vi "IOS_Ephys_GCaMP_WhiskerTracking_Master.vi"() -> ()   [LabVIEW 2013]
uses:
  <vilib>/userdefined/High Color/IMAQdx.ctl
  <vilib>/vision/driver/IMAQdx.llb/IMAQdx Acquisition Mode.ctl
  <vilib>/vision/driver/IMAQdx.llb/IMAQdx Camera Control Mode.ctl
  <vilib>/vision/driver/IMAQdx.llb/IMAQdx Buffer Number Mode.ctl
  <vilib>/DAQmx/write.llb/DAQmx Write (Digital Bool 1Line 1Point).vi
  <vilib>/DAQmx/read.llb/DAQmx Read (Analog 1D Wfm NChan NSamp).vi
  <vilib>/DAQmx/write.llb/DAQmx Write (Digital 1D Bool NChan 1Samp 1Line).vi
  <vilib>/DAQmx/create/channels.llb/DAQmx Create Channel (DO-Digital Output).vi
  <vilib>/DAQmx/create/channels.llb/DAQmx Create Channel (CO-Pulse Generation-Frequency).vi
  <vilib>/DAQmx/configure/timing.llb/DAQmx Timing (Implicit).vi
  <vilib>/DAQmx/create/channels.llb/DAQmx Create Channel (AI-Voltage-Basic).vi
  <vilib>/DAQmx/configure/timing.llb/DAQmx Timing (Sample Clock).vi
  <vilib>/DAQmx/configure/trigger.llb/DAQmx Start Trigger (Digital Edge).vi
  <vilib>/DAQmx/miscellaneous.llb/DAQmx Fill In Error Info.vi
  <vilib>/vision/driver/NI_Vision_Acquisition_Software.lvlib
  <resource>/objmgr/imaqdx.rc
panel:
  in  "Exposure\nTime (microsec)":string="10000"
  out "Dropped Frame Table":string[][](table)
  out "Solenoids":bool[](array[boolean])
  out "Whisker Camera":bool
  out "Analog Data":bool
  out "Analog acquisition length":i32
  in  "Channel Labels":string[](array[string])=["Electrophysiology", "ForceSensor", "Solenoid_LeftPad", "Solenoid_RightPad", "Solenoid_Tail", "Solenoid_Auditory"]
  in  "physical channels":tag="Dev1/ai0:5, Dev1/ai7"
  in  "Whisker Cam ID":T1="cam2"
  in  "WebCam ID":T1="cam1"
  in  "Analog Acquisition Setup":cluster{"Analog Sampling Rate":u16}={"Analog Sampling Rate"=20000} {"Analog Sampling Rate" format="%0.0f"}
  in  "Camera Acquisition Setup":T2={"CBVCam Rate"=30, "WhiskerCam Rate"=150, "WebCam Rate"=15}
  out "Notes Size":i32=7
  out "Notes Reversed":string[](array[string])=["Experimenter", "Animal ID", "Imaged Hemisphere", "Solenoid Pressure", "Isoflurane time", "Session ID", "Amplifier Gain"]
  out "Notes Array":string[](array[string])=["Amplifier Gain", "Session ID", "Isoflurane time", "Solenoid Pressure", "Imaged Hemisphere", "Animal ID", "Experimenter"]
  in  "Session Notes:":T3={"Experimenter"="Kevin", "Animal ID"="T31", "Imaged Hemisphere"="Both", "Solenoid Pressure"="10", "Isoflurane time"="1200", "Session ID"="Habit1", "Amplifier Gain"="10000"}
  in  "Whisker Cam\nTrigger Source":tag="Dev1/ctr1"
  in  "CBV Cam\nTrigger Source":tag="Dev1/ctr0"
  in  "Left Pad":tag="Dev1/port0/line1"
  in  "Right Pad":tag="Dev1/port0/line0"
  in  "Auditory":tag="Dev1/port0/line3"
  in  "Tail":tag="Dev1/port0/line2"
  in  "Stim \nOffset (s)":dbl=15.0
  in  "Stim \nDuration (s)":dbl=0.1 step=0.1
  in  "Inter-Stim\nInterval (s)":dbl=30.0
  in  "Left Pad":dbl=1.0
  in  "Right Pad":dbl=1.0
  in  "Auditory":dbl
  in  "Tail":dbl
  in  "Target Path":path=path "A:/Turner Habituation" caption="Final saved file location"
  out "Dropped":u32(slide)=4 caption="Dropped Whisker\nCamera Frames" scale=0.0..50.0
  out "Current file name":string="170828_12_37_58"
  out "Actual WebCam Frame Rate":dbl(knob) scale=0.0..30.0
  out "WebCam":T4(plugin-control)
  out "CBV Camera":bool=TRUE
  out "Trial Time Elapsed (Min)":cluster{dbl, dbl}(slide)={0.5, 0.05364406000000001} scale=0.0..5.0
  in  "Recording Time (min)":dbl(knob)=5.0 min=0.5 max=10.0 step=0.5 scale=0.0..5.0 scale format="%#_2g"
  in  "Temp Path":path=path "C:/LabView Test Files" caption="Temporary path for\nstreamed data"
  out "Last CBV\nBuffer":i32=97
  in  "Stop":bool
  out "Actual CBVCam\nFrame Rate":dbl(knob)=30.019685039370078 scale=0.0..100.0
  out "Last Whisk\nBuffer":u32=488
  out "Actual WhiskCam\nFrame Rate":dbl(knob)=148.05583250249254 scale=0.0..300.0
  # "Dropped\nIndex"
  # "# Dropped"
  # "File Settings:"
  # "Right Pad"
  # "Left Pad"
  # "Tail"
  # "Auditory"
  # "Stimulation Settings:"
  # "Stim. Ratios:"
  # "Output Channels:"
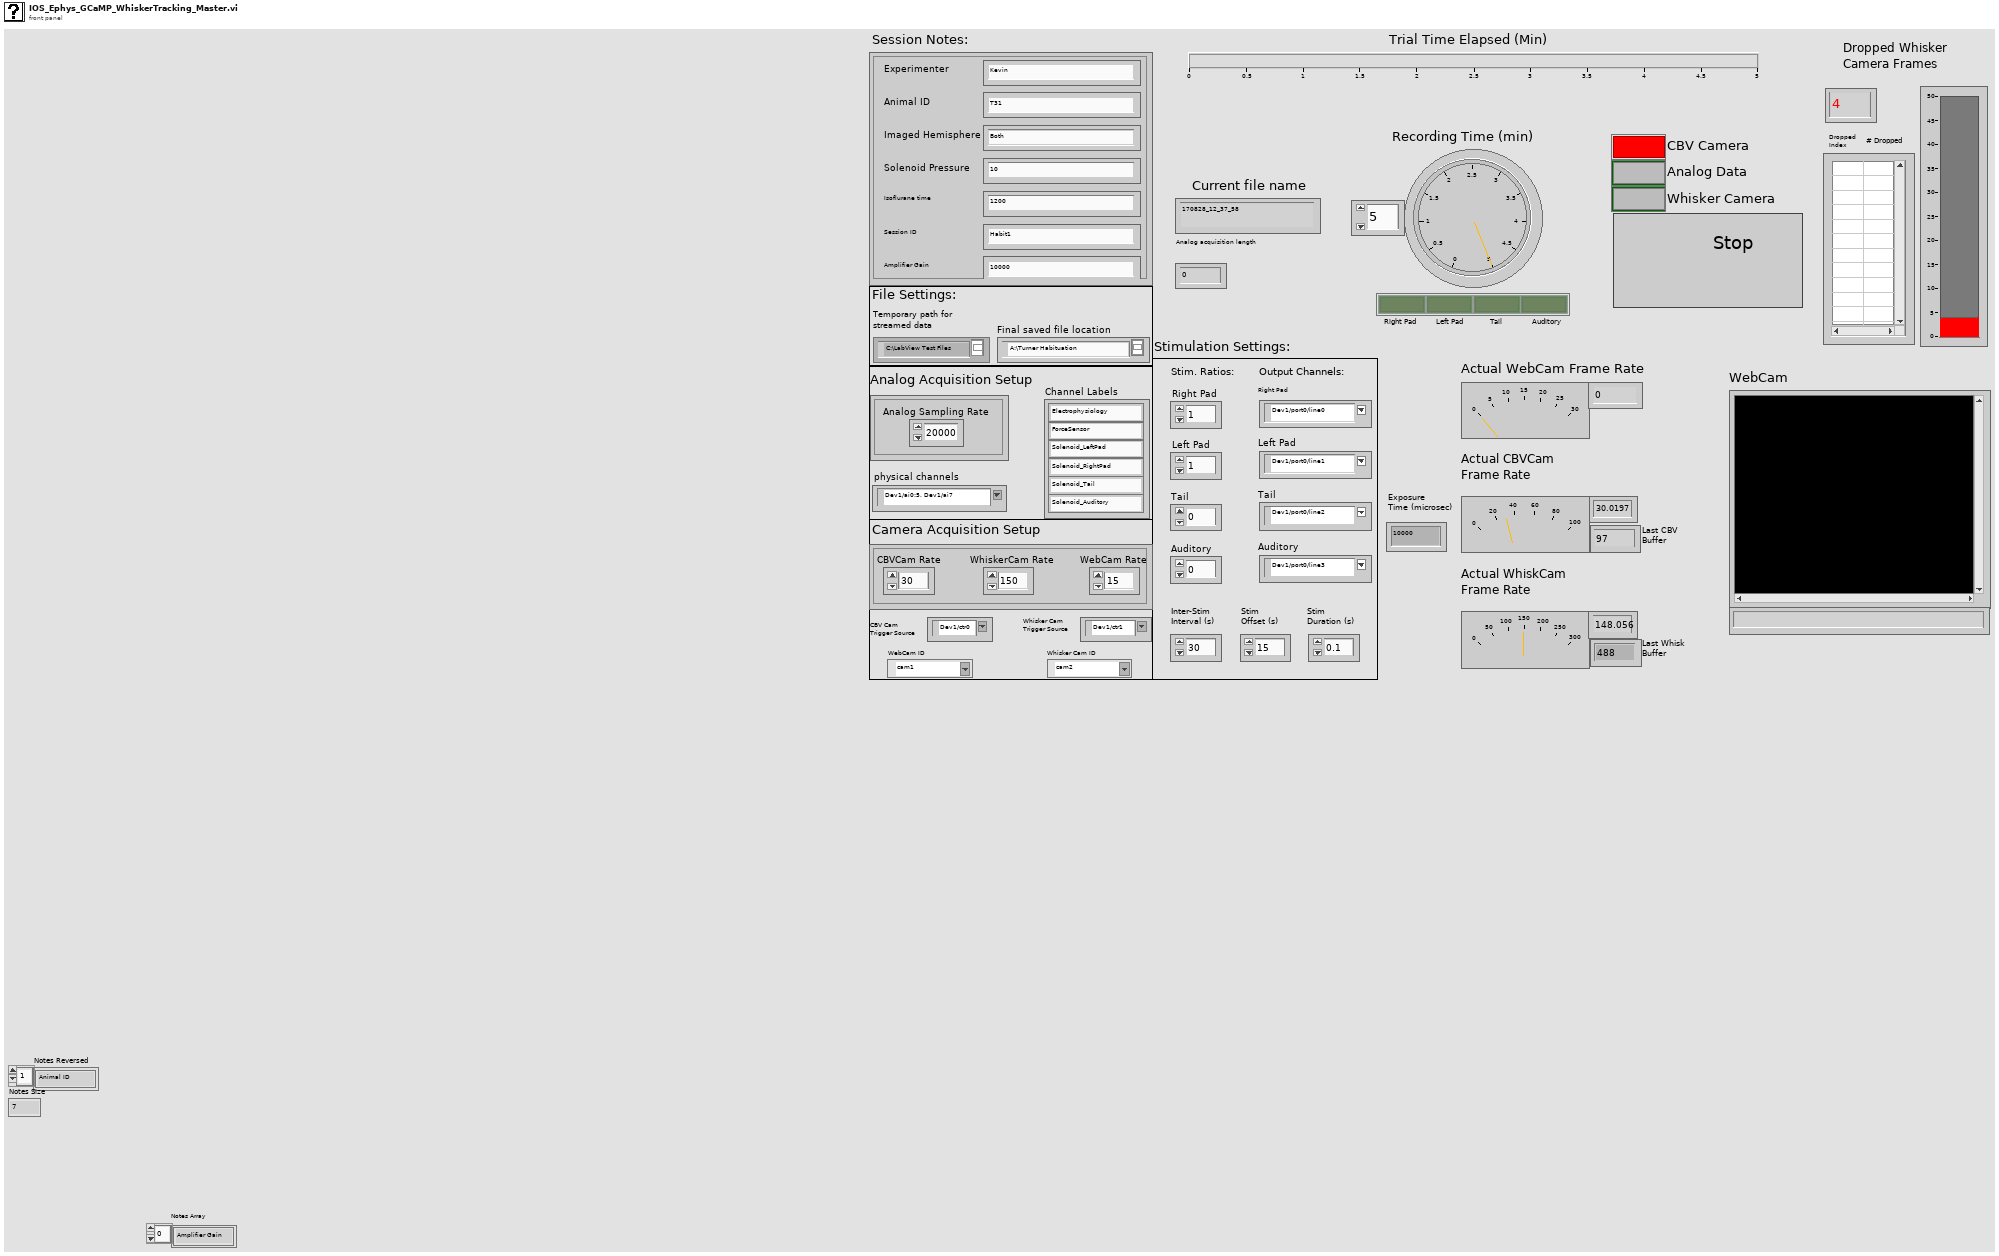
[diagram p1: front panel]
types:
  T1 = typedef "IMAQdx.ctl" = refnum<k21>
  T2 = cluster{"CBVCam Rate":u16, "WhiskerCam Rate":u16, "WebCam Rate":u16}
  T3 = cluster{"Experimenter":string, "Animal ID":string, "Imaged Hemisphere":string, "Solenoid Pressure":string, "Isoflurane time":string, "Session ID":string, "Amplifier Gain":string}
  T4 = typedef "IMAQ Image.ctl" = refnum<image>
  T5 = enum16{"open", "open or create", "create or replace", "create", "open (read-only)"}
  T6 = typedef "Image Type" = u32
  T7 = typedef "NI_Vision_Acquisition_Software.lvlib/IMAQdx Camera Control Mode.ctl" = enum32{"Controller", "Listener"}
  T8 = enum16{"open", "replace", "create", "open or create", "replace or create", "replace or create with confirmation"}
  T9 = typedef "NI_Vision_Acquisition_Software.lvlib/IMAQdx Acquisition Mode.ctl" = enum32{"One Shot", "Continuous"}
  T10 = typedef "IMAQ AVI2 Refnum.ctl" = refnum<k20>
  T11 = enum16{"big-endian, network order", "native, host order", "little-endian"}
  T12 = typedef "NI_Vision_Acquisition_Software.lvlib/IMAQdx Buffer Number Mode.ctl" = enum32{"Next", "Last", "Buffer Number"}
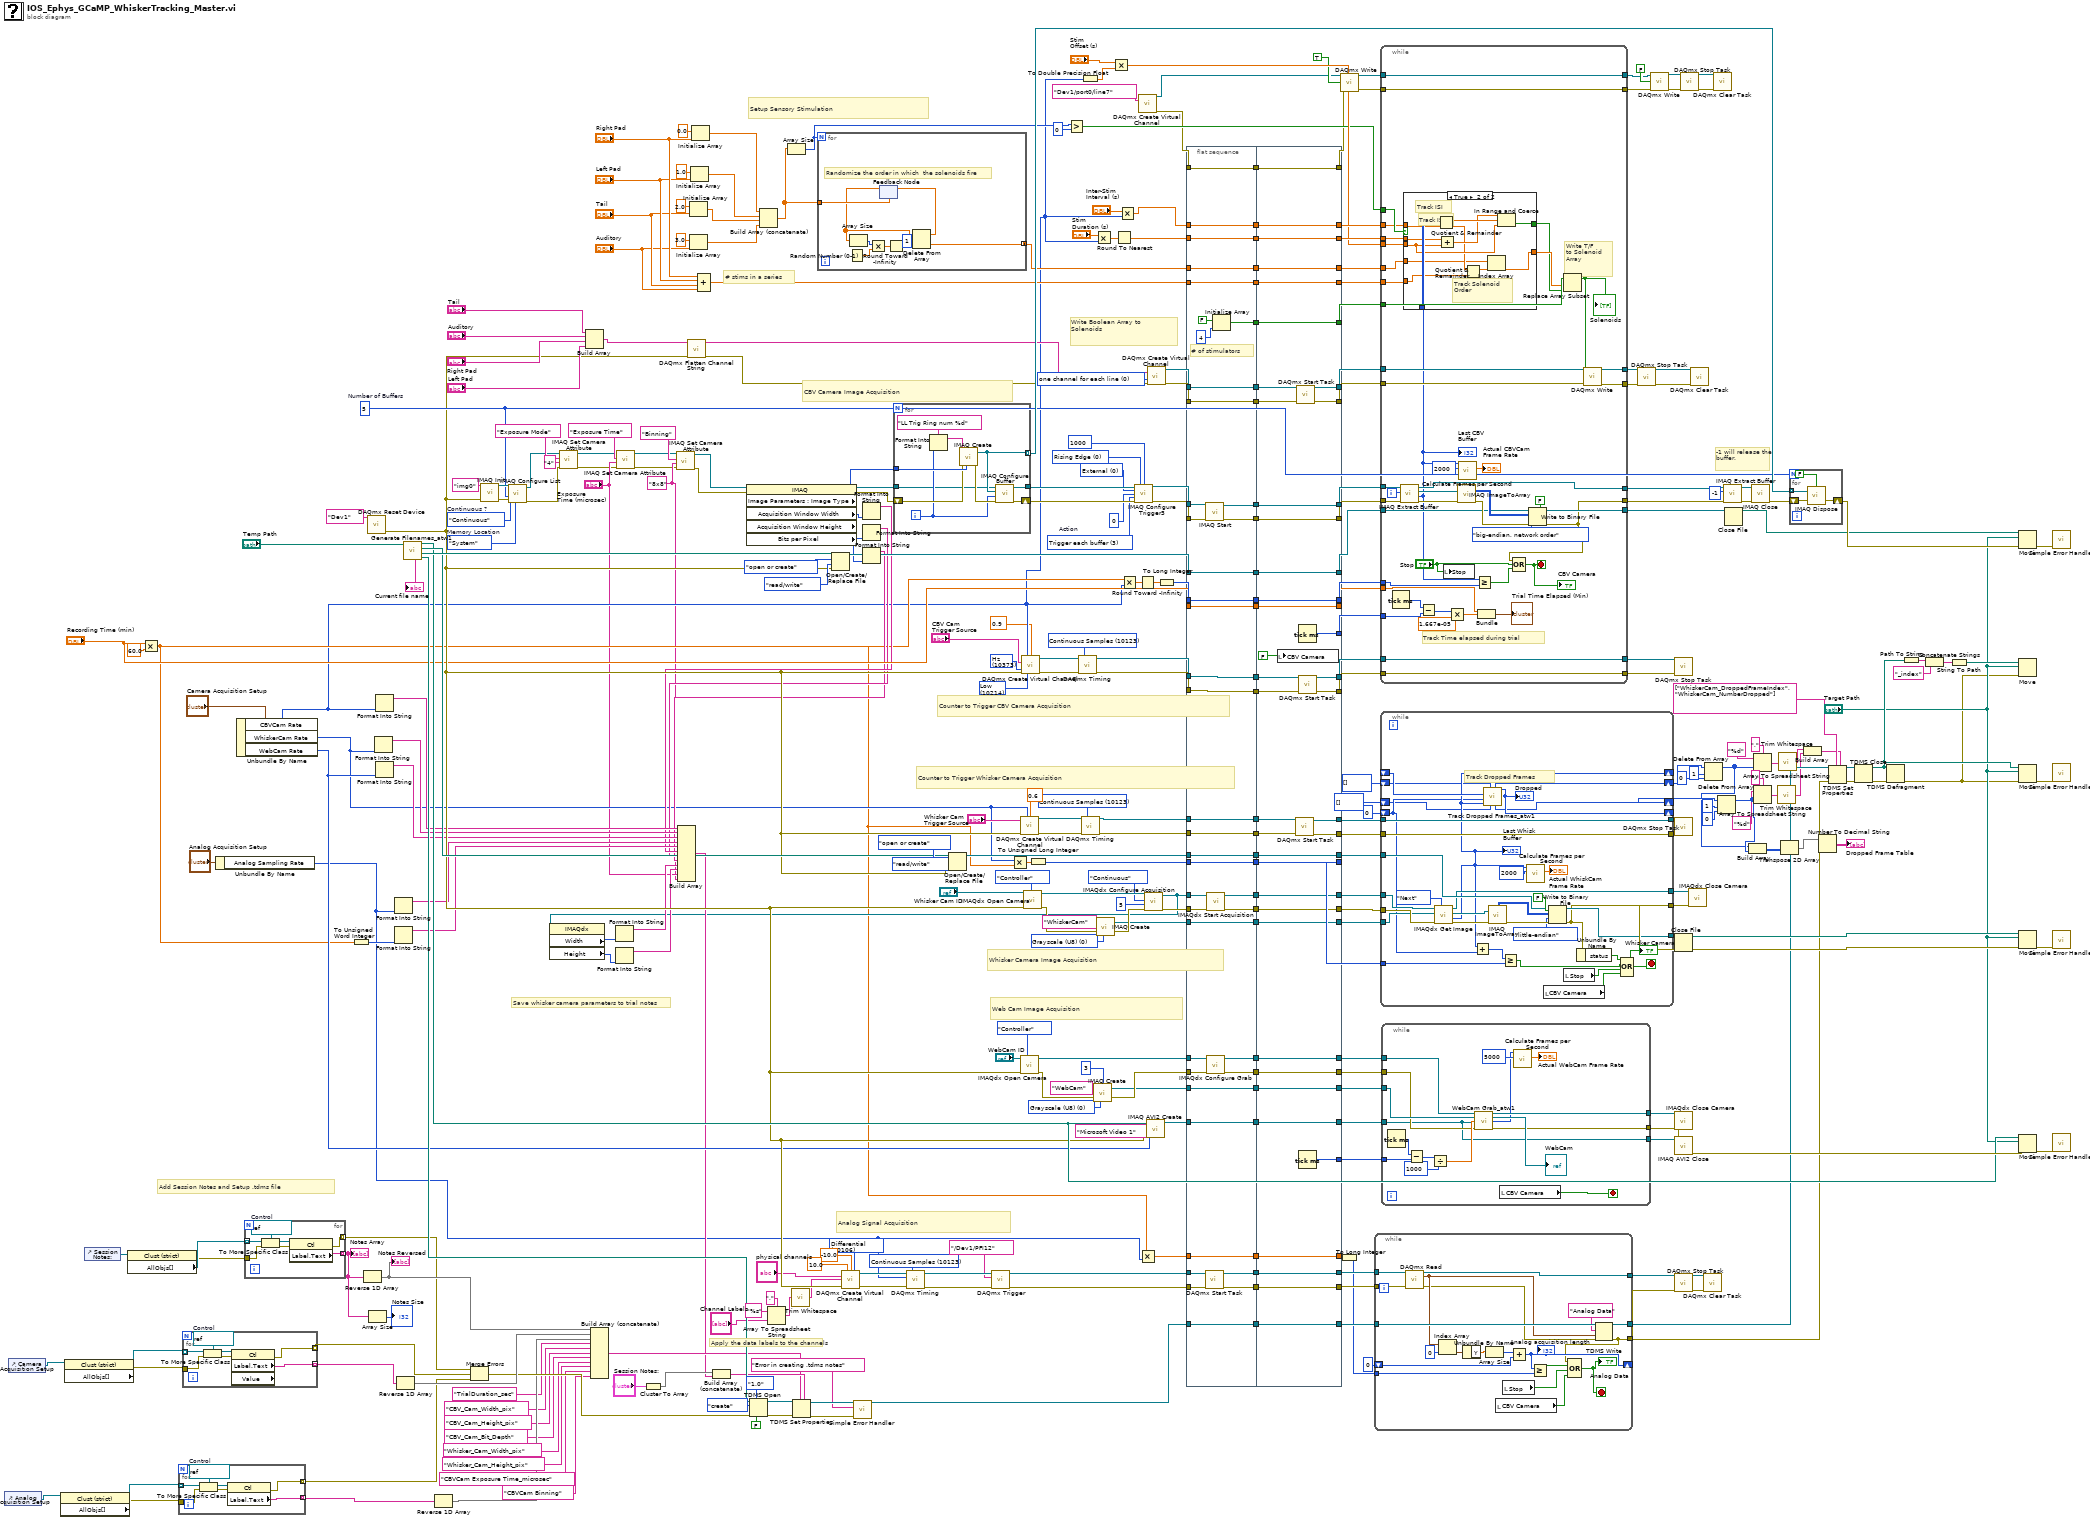
[diagram p0: block diagram]
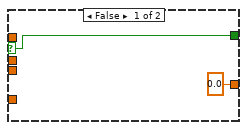
[diagram p2: hidden frame]
diagram:
  w15 = "8x8" ("Attribute Value")
  w189 = 0 items=["one channel for each line", "one channel for all lines"] ("line grouping")
  w248 = 10123 items=["Finite Samples"=10178, "Continuous Samples"=10123, "Hardware Timed Single Point"=12522] ("sample mode")
  w251 = 10106 items=["default"=-1, "RSE"=10083, "NRSE"=10078, "Differential"=10106, "Pseudodifferential"=12529] ("input terminal configuration")
  w305 = T6 0 items=["Grayscale (U8)", "Grayscale (I16)", "Grayscale (SGL)", "Complex (CSG)", "RGB (U32)", "HSL (U32)", "RGB (U64)", "Grayscale (U16)"] ("Image Type")
  w327 = u32 0 items=["Rising Edge", "Falling Edge"] ("Trigger Polarity")
  w330 = u32 0 items=["External"=0, "RTSI"=1, "ISO In"=2, "Scaled Encoder"=5] ("Trigger Type")
  w321 = 10123 items=["Finite Samples"=10178, "Continuous Samples"=10123, "Hardware Timed Single Point"=12522] ("sample mode")
  w324 = 10373 items=["Hz"=10373] ("units")
  w325 = 10214 items=["High"=10192, "Low"=10214] ("idle state")
  w156 = u32 5  # Number of Buffers
  w328 = u32 3 items=["Disabled", "Trigger start of acquisition", "Trigger start of each buffer list", "Trigger each buffer", "Trigger each line (linescan)", "Trigger end of acquisition"]  # Action
  w335 = enum16{"System", "Onboard"}."System"  # Memory Location
  w334 = enum16{"One-Shot", "Continuous"}."Continuous"  # Continuous ?
  w343 = 10123 items=["Finite Samples"=10178, "Continuous Samples"=10123, "Hardware Timed Single Point"=12522] ("sample mode")
  w350 = T6 0 items=["Grayscale (U8)", "Grayscale (I16)", "Grayscale (SGL)", "Complex (CSG)", "RGB (U32)", "HSL (U32)", "RGB (U64)", "Grayscale (U16)"] ("Image Type")
  # "Save whisker camera parameters to trial notes"
  # "Apply the data labels to the channels"
  # "Setup Sensory Stimulation"
  # "CBV Camera Image Acquisition"
  # "Counter to Trigger CBV Camera Acquisition"
  # "Counter to Trigger Whisker Camera Acquisition"
  # "Whisker Camera Image Acquisition"
  # "Web Cam Image Acquisition"
  # "Add Session Notes and Setup .tdms file"
  # "Analog Signal Acquisition"
  # "Write Boolean Array to \nSolenoids"
  # "# stims in a series"
  # "-1 will release the buffer."
  n1 = control-ref of="Analog Acquisition Setup"() -> (w116:refnum<vi>)
  n2 = control-ref of="Camera Acquisition Setup"() -> (w117:refnum<vi>)
  n3 = property class="Clust (strict)"(reference=w116) -> (error out=w114:errorcluster, "AllObjs[]"=w115:refnum<vi>[])  [unwired: 1 in, 1 out]
  n4 = property class="Clust (strict)"(reference=w117) -> (error out=w139:errorcluster, "AllObjs[]"=w138:refnum<vi>[])  [unwired: 1 in, 1 out]
  n5 = control-ref of="Session Notes:"() -> (w142:refnum<vi>)
  n6 = property class="Clust (strict)"(reference=w142) -> (error out=w145:errorcluster, "AllObjs[]"=w146:refnum<vi>[])  [unwired: 1 in, 1 out]
  n7 = Multiply(x="Recording Time (min)", y=60.0) -> (x*y=w49:dbl)
  n8 = for {
    tunnel: [w362] -> w112 mode=indexing
    tunnel: w115 -> [w361] mode=indexing
    tunnel: w114 -> [w360]
    tunnel: [w358] -> w113 mode=indexing
    w363 = refnum<vi> refnum  # Control
    n9 = To More Specific Class(target class=w363, reference=w361, error in=w360) -> (specific class reference=w364:refnum<vi>, error out=w359:errorcluster)
    n10 = property class="Ctl"(reference=w364, error in=w359) -> (error out=w358:errorcluster, "Label.Text"=w362:string)  [unwired: 1 out]
  }
  n11 = for {
    tunnel: [w369] -> w140 mode=indexing
    tunnel: w138 -> [w368] mode=indexing
    tunnel: w139 -> [w367]
    tunnel: [w365] -> w123 mode=indexing
    w370 = refnum<vi> refnum  # Control
    n12 = To More Specific Class(target class=w370, reference=w368, error in=w367) -> (specific class reference=w371:refnum<vi>, error out=w366:errorcluster)
    n13 = property class="Ctl" props=["Label", "Text", "Value"](reference=w371, error in=w366) -> (error out=w365:errorcluster, "Label.Text"=w369:string)  [unwired: 2 out]
  }
  n14 = Unbundle By Name("Analog Acquisition Setup") -> ("Analog Sampling Rate"=w55:u16)
  n15 = Unbundle By Name("Camera Acquisition Setup") -> ("CBVCam Rate"=w23:u16, "WhiskerCam Rate"=w50:u16, "WebCam Rate"=w109:u16)
  n16 = for {
    tunnel: [w376] -> w144 mode=indexing
    tunnel: w146 -> [w375] mode=indexing
    tunnel: w145 -> [w374]
    tunnel: [w372] -> w124 mode=indexing
    w377 = refnum<vi> refnum  # Control
    n17 = To More Specific Class(target class=w377, reference=w375, error in=w374) -> (specific class reference=w378:refnum<vi>, error out=w373:errorcluster)
    n18 = property class="Ctl"(reference=w378, error in=w373) -> (error out=w372:errorcluster, "Label.Text"=w376:string)  [unwired: 1 out]
  }
  "Notes Array" <- w144
  n19 = To Unsigned Word Integer(number=w49) -> (unsigned 16bit integer=w91:u16)
  n20 = Reverse 1D Array(array=w144) -> (reversed array=w129:string[])
  "Notes Reversed" <- w129
  n21 = call <vilib>:"DAQmx Reset Device.vi"("device in"=tag "Dev1") -> ("error out"=w141:errorcluster)  [unwired: 14 in]
  n22 = Array Size(array=w144) -> (size(s)=→"Notes Size":i32)
  n23 = Format Into String(w50) -> (resulting string=w107:string)  [unwired: 3 in, 1 out]
  n24 = Format Into String(w23) -> (resulting string=w108:string)  [unwired: 3 in, 1 out]
  n25 = Format Into String(w109) -> (resulting string=w106:string)  [unwired: 3 in, 1 out]
  n26 = Format Into String(w55) -> (resulting string=w105:string)  [unwired: 3 in, 1 out]
  n27 = Format Into String(w91) -> (resulting string=w93:string)  [unwired: 3 in, 1 out]
  n28 = Reverse 1D Array(array=w140) -> (reversed array=w128:string[])
  n29 = call "Generate Filenames_atw1.vi"("path"="Temp Path") -> ("TDMS Path"=w135:path, "Dalsa Path"=w313:path, "Basler Path"=w308:path, "WebCam Path"=w213:path, "Analog file name"=→"Current file name":string)  [unwired: 5 in, 1 out]
  n30 = Reverse 1D Array(array=w112) -> (reversed array=w111:string[])
  n31 = Merge Errors(w124, w123, w113) -> (w122:errorcluster)
  n32 = call <vilib>:"IMAQ Init.vi"("error in (no error)"=w141, "Interface Name"="img0") -> ("error out"=w341:errorcluster, "IMAQ Session Out"=w342:refnum<k11>)  [unwired: 8 out]
  n33 = call <vilib>:"IMAQ Configure List.vi"("Memory Location"=w335, "error in (no error)"=w341, "Number of buffers"=w156, "Continuous?"=w334, "IMAQ Session In"=w342) -> ("error out"=w14:errorcluster, "IMAQ Session Out"=w10:refnum<k11>)  [unwired: 1 in, 4 out]
  n34 = call <vilib>:"IMAQ Set Camera Attribute.vi"("error in (no error)"=w14, "Attribute Value"="4", "Camera Attribute"="Exposure Mode", "IMAQ Session In"=w10) -> ("error out"=w13:errorcluster, "IMAQ Session Out"=w9:refnum<k11>)  [unwired: 4 in]
  n35 = Build Array("Tail", "Auditory", "Right Pad", "Left Pad") -> (w148:tag[])
  n36 = Build Array (concatenate)(w129, w128, w111, "TrialDuration_sec", "CBV_Cam_Width_pix", "CBV_Cam_Height_pix", "CBV_Cam_Bit_Depth", "Whisker_Cam_Width_pix", "Whisker_Cam_Height_pix", "CBVCam Exposure Time_microsec" ("element"), "CBVCam Binning" ("element")) -> (w126:string[])
  n37 = call <vilib>:"IMAQ Set Camera Attribute.vi"("error in (no error)"=w13, "Attribute Value"="Exposure\nTime (microsec)", "Camera Attribute"="Exposure Time", "IMAQ Session In"=w9) -> ("error out"=w12:errorcluster, "IMAQ Session Out"=w8:refnum<k11>)  [unwired: 4 in]
  n38 = Cluster To Array(cluster="Session Notes:") -> (array=w136:string[])
  n39 = call <vilib>:"IMAQ Set Camera Attribute.vi"("error in (no error)"=w12, "Attribute Value"=w15, "Camera Attribute"="Binning", "IMAQ Session In"=w8) -> ("error out"=w11:errorcluster, "IMAQ Session Out"=w7:refnum<k11>)  [unwired: 4 in]
  n40 = call <vilib>:"DAQmx Flatten Channel String.vi"("names in"=w148, "error in"=w141) -> ("names out"=w153:string, "error out"=w147:errorcluster)  [unwired: 12 in]
  n41 = Initialize Array(2.0 ("element"), "Tail") -> (w194:dbl[])
  n42 = Initialize Array(3.0 ("element"), "Auditory") -> (w193:dbl[])
  n43 = Initialize Array(1.0 ("element"), "Left Pad") -> (w195:dbl[])
  n44 = Initialize Array(0.0 ("element"), "Right Pad") -> (w196:dbl[])
  n45 = Compound Arithmetic op=ADD("Right Pad", "Left Pad", "Tail", "Auditory") -> (w173:dbl)
  n46 = property class="IMAQ"(reference=w7, error in=w11) -> (reference out=w25:refnum<k11>, error out=w24:errorcluster, "Image Parameters : Image Type"=w336:u32, "Acquisition Window Width"=w88:u32, "Acquisition Window Height"=w87:u32, "Bits per Pixel"=w86:u32)
  n47 = TDMS Open(6:FALSE ("disable buffering? (T)"), 7:enum16{"1.0", "2.0"}."1.0" ("file format version (2.0)"), 8:w122, 10:T5."create" ("operation (0:open)"), 11:w135) -> (0:w130:errorcluster, 3:w131:refnum<k34>)  [unwired: 2 in]
  n48 = Build Array (concatenate)(w196, w195, w194, w193) -> (w192:dbl[])
  n49 = Array To Spreadsheet String(delimiter (Tab)=",", array="Channel Labels", 3:"%s" ("format string")) -> (spreadsheet string=w97:string)
  n50 = Array Size(array=w192) -> (size(s)=w102:i32)
  n51 = call <vilib>:"Trim Whitespace.vi"("string"=w97) -> ("trimmed string"=w96:string)  [unwired: 1 in]
  n52 = for {
    N: w102 -> [_]
    tunnel: w192 -> [w382]
    tunnel: [w379] -> w170 mode=concatenating
    # "Randomize the order in which  the solenoids fire"
    n53 = Random Number (0-1)() -> (number: 0 to 1=w386:dbl)
    n54 = feedback #1(w382) -> (w381:dbl[])
    n55 = Array Size(array=w381) -> (size(s)=w387:i32)
    n56 = Multiply(x=w387, y=w386) -> (x*y=w385:dbl)
    n57 = Round Toward -Infinity(1:w385) -> (0:w384:dbl)
    n58 = Delete From Array(array=w381, length=1, index=w384) -> (deleted portion=w379:dbl[], array with subset deleted=w380:dbl[])
    n59 = feedback-in #1(w380) -> ()
  }
  n60 = Open/Create/Replace File(file path (use dialog)=w313, error in=w141, operation (0:open)=T8."open or create", access (0:read/write)=enum16{"read/write", "read-only", "write-only"}."read/write") -> (refnum out=w252:refnum<file>)  [unwired: 2 in, 2 out]
  n61 = call-poly <vilib>:"DAQmx Create Virtual Channel.vi"("maximum value"=10.0, "minimum value"=-10.0, "input terminal configuration"=w251, "physical channels"="physical channels", "name to assign"=w96, "error in"=w141) -> ("task out"=w250:refnum<k21>, "error out"=w249:errorcluster)  [unwired: 8 in]
  n62 = Format Into String(w88) -> (resulting string=w85:string)  [unwired: 3 in, 1 out]
  n63 = Format Into String(w87) -> (resulting string=w84:string)  [unwired: 3 in, 1 out]
  n64 = Format Into String(w86) -> (resulting string=w83:string)  [unwired: 3 in, 1 out]
  n65 = for {
    N: w156 -> [_]
    tunnel: [w397] -> w332
    tunnel: w336 -> [w395]
    shift-right: [w396] -> w331
    shift-left: w24 -> [w394]
    tunnel: [w389] -> w333 mode=indexing
    tunnel: w25 -> [w388]
    i -> [w390]
    n66 = Format Into String(format string="LL Trig Ring num %d", w390) -> (resulting string=w392:string)  [unwired: 2 in, 1 out]
    n67 = call "IMAQ Create"("Image Name"=w392, "Image Type"=w395, "error in (no error)"=w394) -> ("New Image"=w389:T4, "error out"=w393:errorcluster)  [unwired: 1 in, 1 out]
    n68 = call <vilib>:"IMAQ Configure Buffer.vi"("error in (no error)"=w393, "Buffer Number"=w390, "Image In"=w389, "IMAQ Session In"=w388) -> ("error out"=w396:errorcluster, "IMAQ Session Out"=w397:refnum<k11>)  [unwired: 2 in, 4 out]
  }
  n69 = call-poly <vilib>:"DAQmx Timing.vi"("task/channels in"=w250, "sample mode"=w248, "rate"=w55, "error in"=w249) -> ("task out"=w247:refnum<k21>, "error out"=w246:errorcluster)  [unwired: 10 in]
  n70 = Open/Create/Replace File(file path (use dialog)=w308, error in=w141, operation (0:open)=T8."open or create", access (0:read/write)=enum16{"read/write", "read-only", "write-only"}."read/write") -> (refnum out=w271:refnum<file>)  [unwired: 2 in, 2 out]
  n71 = call-poly <vilib>:"DAQmx Trigger.vi"("task/channels in"=w247, "source"=tag "/Dev1/PFI12", "error in"=w246) -> ("task out"=w244:refnum<k21>, "error out"=w243:errorcluster)  [unwired: 11 in]
  n72 = Multiply(x=w50, y=w49) -> (x*y=w48:dbl)
  n73 = call <vilib>:"IMAQdx Open Camera.vi"("Camera Control Mode"=IMAQdx_Camera_Control_Mode."Controller", "error in"=w141, "Session In"="WebCam ID") -> ("error out"=w301:errorcluster, "Session Out"=w299:T1)  [unwired: 7 in]
  n74 = call-poly <vilib>:"DAQmx Create Virtual Channel.vi"("frequency"=w50, "duty cycle"=0.6, "counter"="Whisker Cam\nTrigger Source", "error in"=w141) -> ("task out"=w345:refnum<k21>, "error out"=w344:errorcluster)  [unwired: 10 in]
  n75 = call-poly <vilib>:"DAQmx Create Virtual Channel.vi"("frequency"=w23, "duty cycle"=0.9, "counter"="CBV Cam\nTrigger Source", "units"=w324, "error in"=w141, "idle state"=w325) -> ("task out"=w323:refnum<k21>, "error out"=w322:errorcluster)  [unwired: 8 in]
  n76 = call <vilib>:"IMAQdx Open Camera.vi"("Camera Control Mode"=IMAQdx_Camera_Control_Mode."Controller", "error in"=w141, "Session In"="Whisker Cam ID") -> ("error out"=w353:errorcluster, "Session Out"=w356:T1)  [unwired: 7 in]
  n77 = To Unsigned Long Integer(number=w48) -> (unsigned 32bit integer=w47:u32)
  n78 = Greater?(x=w102, y=0) -> (0:w100:bool)
  n79 = call-poly <vilib>:"DAQmx Timing.vi"("task/channels in"=w323, "sample mode"=w321, "error in"=w322) -> ("task out"=w234:refnum<k21>, "error out"=w232:errorcluster)  [unwired: 11 in]
  n80 = call-poly <vilib>:"DAQmx Timing.vi"("task/channels in"=w345, "sample mode"=w343, "error in"=w344) -> ("task out"=w230:refnum<k21>, "error out"=w228:errorcluster)  [unwired: 11 in]
  n81 = To Double Precision Float(number=w23) -> (double precision float=w154:dbl)
  n82 = call "IMAQ Create"("Border Size"=3, "Image Name"="WebCam", "Image Type"=w305, "error in (no error)"=w301) -> ("New Image"=w298:T4, "error out"=w300:errorcluster)  [unwired: 1 in]
  n83 = Multiply(x="Stim \nDuration (s)", y=w23) -> (x*y=w164:dbl)
  n84 = call "IMAQ Create"("Image Name"="WhiskerCam", "Image Type"=w350, "error in (no error)"=w353) -> ("New Image"=w73:T4, "error out"=w351:errorcluster)  [unwired: 2 in]
  n85 = Multiply(x="Stim \nOffset (s)", y=w154) -> (x*y=w155:dbl)
  n86 = Round To Nearest(number=w164) -> (nearest integer value=w163:dbl)
  n87 = Multiply(x="Inter-Stim\nInterval (s)", y=w23) -> (x*y=w177:dbl)
  n88 = Multiply(x=w49, y=w23) -> (x*y=w310:dbl)
  n89 = call <vilib>:"IMAQ Configure Trigger3.vi"("IMAQ Session In"=w332, "Polarity"=w327, "Frame timeout (ms)"=u32 1000 ("Frame Timeout (ms)"), "Type"=w330, "Line Number"=u32 0 ("Trigger Line Number"), "Action"=w328, "error in (no error)"=w331) -> ("IMAQ Session Out"=w270:refnum<k11>, "error out"=w269:errorcluster)  [unwired: 2 in, 5 out]
  n90 = call-poly <vilib>:"DAQmx Create Virtual Channel.vi"("lines"=tag "Dev1/port0/line7") -> ("task out"=w39:refnum<k21>, "error out"=w42:errorcluster)  [unwired: 13 in]
  n91 = Round Toward -Infinity(1:w310) -> (0:w309:dbl)
  n92 = Multiply(x=w49, y=w55) -> (x*y=w54:dbl)
  n93 = call <vilib>:"IMAQdx Configure Acquisition.vi"("error in"=w351, "Number of Buffers"=u32 5, "Continuous?"=IMAQdx_Acquisition_Mode."Continuous", "Session In"=w356) -> ("error out"=w280:errorcluster, "Session Out"=w74:T1)  [unwired: 6 in]
  n94 = property class="IMAQdx"(reference=w74) -> ("Width"=w90:u32, "Height"=w89:u32)  [unwired: 1 in, 2 out]
  n95 = Format Into String(w90) -> (resulting string=w82:string)  [unwired: 3 in, 1 out]
  n96 = Format Into String(w89) -> (resulting string=w81:string)  [unwired: 3 in, 1 out]
  n97 = Build Array(w108, w107, w106, w105, w93, w85, w84, w83, w82, w81, "Exposure\nTime (microsec)", w15) -> (w104:string[])
  n98 = Build Array (concatenate)(w136, w104) -> (w127:string[])
  n99 = TDMS Set Properties(5:w127, 7:w126, 8:w130, 11:w131) -> (0:w121:errorcluster, 3:w125:refnum<k34>)  [unwired: 2 in, 2 out]
  n100 = call <vilib>:"Simple Error Handler.vi"("error source (\" \")"="Error in creating .tdms notes" ("error source (\" \")"), "error in (no error)"=w121) -> ()  [unwired: 3 in, 5 out]
  n101 = call "IMAQ AVI2 Create"("error in (no error)"=w141, "Codec"="Microsoft Video 1", "Frames Per Second"=w109, "AVI Path"=w213) -> ("AVI Refnum"=w291:T10)  [unwired: 6 in, 1 out]
  n102 = call-poly <vilib>:"DAQmx Create Virtual Channel.vi"("lines"=w153, "line grouping"=w189, "error in"=w147) -> ("task out"=w187:refnum<k21>, "error out"=w185:errorcluster)  [unwired: 11 in]
  n103 = To Long Integer(number=w309) -> (32bit integer=w259:i32)
  n104 = flat-sequence {
    tunnel: w300 -> [w437]
    tunnel: w299 -> [w436]
    tunnel: w298 -> [w435]
    tunnel: [w435] -> w297
    tunnel: [w434] -> w295
    tunnel: [w433] -> w293
    tunnel: w291 -> [w432]
    tunnel: [w432] -> w290
    tunnel: w74 -> [w431]
    tunnel: w280 -> [w430]
    tunnel: [w429] -> w278
    tunnel: [w428] -> w276
    tunnel: [w427] -> w274
    tunnel: w73 -> [w427]
    tunnel: [w426] -> w272
    tunnel: w271 -> [w426]
    tunnel: w270 -> [w425]
    tunnel: w269 -> [w424]
    tunnel: [w423] -> w267
    tunnel: [w422] -> w265
    tunnel: w259 -> [w421]
    tunnel: [w421] -> w258
    tunnel: "Recording Time (min)" -> [w420]
    tunnel: [w420] -> w255
    tunnel: [w419] -> w253
    tunnel: w252 -> [w419]
    tunnel: w244 -> [w418]
    tunnel: w243 -> [w417]
    tunnel: [w416] -> w242
    tunnel: [w415] -> w241
    tunnel: [w414] -> w236
    tunnel: w125 -> [w414]
    tunnel: w234 -> [w413]
    tunnel: [w413] -> w233
    tunnel: w232 -> [w412]
    tunnel: [w412] -> w231
    tunnel: w230 -> [w411]
    tunnel: [w411] -> w229
    tunnel: w228 -> [w410]
    tunnel: [w410] -> w227
    tunnel: w187 -> [w409]
    tunnel: [w409] -> w188
    tunnel: w185 -> [w408]
    tunnel: [w408] -> w186
    tunnel: w177 -> [w407]
    tunnel: [w407] -> w176
    tunnel: [w406] -> w174
    tunnel: w163 -> [w406]
    tunnel: w173 -> [w405]
    tunnel: [w405] -> w172
    tunnel: w170 -> [w404]
    tunnel: [w404] -> w169
    tunnel: [w402] -> w167
    tunnel: w54 -> [w400]
    tunnel: [w400] -> w53
    tunnel: w47 -> [w399]
    tunnel: [w399] -> w46
    tunnel: w42 -> [w398]
    tunnel: [w398] -> w41
    tunnel: [w476] -> w302
    tunnel: w297 -> [w475]
    tunnel: [w475] -> w296
    tunnel: w295 -> [w474]
    tunnel: [w474] -> w294
    tunnel: w293 -> [w473]
    tunnel: [w473] -> w292
    tunnel: w290 -> [w472]
    tunnel: [w472] -> w289
    tunnel: [w454] -> w285
    tunnel: [w453] -> w283
    tunnel: [w471] -> w279
    tunnel: w278 -> [w471]
    tunnel: [w470] -> w277
    tunnel: w276 -> [w470]
    tunnel: [w469] -> w275
    tunnel: w274 -> [w469]
    tunnel: [w468] -> w273
    tunnel: w272 -> [w468]
    tunnel: [w467] -> w268
    tunnel: w267 -> [w467]
    tunnel: [w466] -> w266
    tunnel: w265 -> [w466]
    tunnel: [w458] -> w263
    tunnel: [w457] -> w261
    tunnel: [w465] -> w260
    tunnel: w258 -> [w464]
    tunnel: [w464] -> w257
    tunnel: [w463] -> w256
    tunnel: w255 -> [w463]
    tunnel: [w462] -> w254
    tunnel: w253 -> [w462]
    tunnel: [w461] -> w239
    tunnel: w242 -> [w461]
    tunnel: [w460] -> w240
    tunnel: w241 -> [w460]
    tunnel: [w459] -> w237
    tunnel: w236 -> [w459]
    tunnel: w233 -> [w456]
    tunnel: w231 -> [w455]
    tunnel: w229 -> [w452]
    tunnel: w227 -> [w451]
    tunnel: w188 -> [w450]
    tunnel: w186 -> [w449]
    tunnel: [w448] -> w184
    tunnel: [w447] -> w183
    tunnel: [w446] -> w178
    tunnel: w176 -> [w446]
    tunnel: [w445] -> w175
    tunnel: w174 -> [w445]
    tunnel: w172 -> [w444]
    tunnel: [w444] -> w171
    tunnel: w169 -> [w443]
    tunnel: [w443] -> w168
    tunnel: w167 -> [w442]
    tunnel: [w442] -> w166
    tunnel: w53 -> [w441]
    tunnel: [w441] -> w52
    tunnel: w46 -> [w440]
    tunnel: [w440] -> w45
    tunnel: w41 -> [w439]
    tunnel: [w439] -> w40
    frame #0 {
      # "# of stimulators"
      n105 = call <vilib>:"DAQmx Start Task.vi"("task/channels in"=w418, "error in"=w417) -> ("task out"=w416:refnum<k21>, "error out"=w415:errorcluster)  [unwired: 12 in]
      n106 = call <vilib>:"IMAQ Start.vi"("error in (no error)"=w424, "IMAQ Session In"=w425) -> ("error out"=w422:errorcluster, "IMAQ Session Out"=w423:refnum<k11>)  [unwired: 8 out]
      n107 = call <vilib>:"IMAQdx Configure Grab.vi"("error in"=w437, "Session In"=w436) -> ("error out"=w433:errorcluster, "Session Out"=w434:T1)  [unwired: 8 in]
      n108 = call <vilib>:"IMAQdx Start Acquisition.vi"("error in"=w430, "Session In"=w431) -> ("error out"=w428:errorcluster, "Session Out"=w429:T1)  [unwired: 8 in]
      n109 = Initialize Array(FALSE, 4 ("dimension size")) -> (w402:bool[])
    }
    frame #1 {
      n110 = local write "CBV Camera"(FALSE ("Finished Acquiring")) -> ()
      n111 = call <vilib>:"DAQmx Start Task.vi"("task/channels in"=w452, "error in"=w451) -> ("task out"=w454:refnum<k21>, "error out"=w453:errorcluster)  [unwired: 12 in]
      n112 = call <vilib>:"DAQmx Start Task.vi"("task/channels in"=w450, "error in"=w449) -> ("task out"=w448:refnum<k21>, "error out"=w447:errorcluster)  [unwired: 12 in]
      n113 = Tick Count (ms)() -> (millisecond timer value=w465:u32)
      n114 = call <vilib>:"DAQmx Start Task.vi"("task/channels in"=w456, "error in"=w455) -> ("task out"=w458:refnum<k21>, "error out"=w457:errorcluster)  [unwired: 12 in]
      n115 = Tick Count (ms)() -> (millisecond timer value=w476:u32)
    }
  }
  n116 = To Long Integer(number=w52) -> (32bit integer=w51:i32)
  n117 = call-poly <vilib>:"DAQmx Write.vi"("task/channels in"=w39, "data"=TRUE, "error in"=w40) -> ("task out"=w37:refnum<k21>, "error out"=w35:errorcluster)  [unwired: 10 in, 1 out]
  n118 = while {
    tunnel: w240 -> [w496]
    tunnel: w239 -> [w495]
    tunnel: w237 -> [w494]
    tunnel: [w493] -> w72
    tunnel: [w477] -> w71
    tunnel: [w492] -> w235
    shift-right: [w484] -> _
    shift-left: 0 -> [w485]
    tunnel: w51 -> [w483]
    stop <- w479 stop-if-true
    n119 = call-poly <vilib>:"DAQmx Read.vi"("task/channels in"=w495, "error in"=w496) -> ("task out"=w492:refnum<k21>, "data"=w490:waveform(dbl)[], "error out"=w482:errorcluster)  [unwired: 11 in]
    n120 = Index Array(array=w490, index=0) -> (element=w488:waveform(dbl))
    n121 = Unbundle By Name(w488) -> ("Y"=w487:dbl[])
    n122 = Array Size(array=w487) -> (size(s)=w486:i32)
    n123 = local read "CBV Camera"() -> (w478:bool)
    n124 = local read "Stop"() -> (w480:bool)
    n125 = Add(x=w486, y=w485) -> (x+y=w484:i32)
    "Analog acquisition length" <- w484
    n126 = Greater Or Equal?(x=w484, y=w483) -> (x >= y?=w481:bool)
    n127 = TDMS Write(0:w494, 5:"Analog Data" ("group name in (Untitled)"), 9:w490, 11:w482) -> (4:w493:refnum<k34>, 15:w477:errorcluster)  [unwired: 2 in, 2 out]
    n128 = Compound Arithmetic op=OR(w477, w481, w480, w478) -> (w479:bool)
    "Analog Data" <- w479
  }
  n129 = while {
    tunnel: w285 -> [w519]
    tunnel: [w520] -> w284
    tunnel: w283 -> [w520]
    tunnel: [w519] -> w282
    tunnel: [w508] -> w68
    tunnel: [w509] -> w157
    tunnel: [w518] -> w281
    tunnel: w279 -> [w517]
    tunnel: w277 -> [w516]
    tunnel: w275 -> [w515]
    tunnel: w273 -> [w514]
    shift-right: [w507] -> _
    shift-left: _ -> [w513]
    shift-right: [w512] -> _
    shift-left: u32 0 ("New Lost") -> [w506]
    shift-right: [w511] -> w57
    shift-left: u32[] [] ("NewBuffNum") -> [w497]
    shift-right: [w510] -> w221
    shift-left: u32[] [] ("NewNumLost") -> [w498]
    tunnel: w45 -> [w504]
    stop <- w500 stop-if-true
    # "Track Dropped Frames"
    n130 = call <vilib>:"IMAQdx Get Image.vi"("Buffer Number Mode (Next)"=IMAQdx_Buffer_Number_Mode."Next", "error in"=w516, "Image In"=w515, "Session In"=w517) -> ("error out"=w528:errorcluster, "Buffer Number Out"=w507:u32, "Image Out"=w527:T4, "Session Out"=w508:T1)  [unwired: 4 in]
    "Last Whisk\nBuffer" <- w507
    n131 = Add(x=w507, y=w506) -> (x+y=w505:u32)
    n132 = call "Track Dropped Frames_atw1.vi"("NumLost"=w498, "BuffNum"=w497, "Curr Buffer"=w507, "Prev Lost"=w506, "Prev Buffer"=w513) -> ("New Lost"=w512:u32, "NewNumLost"=w510:u32[], "NewBuffNum"=w511:u32[])  [unwired: 4 in]
    "Dropped" <- w512
    n133 = call "IMAQ ImageToArray"("error in (no error)"=w528, "Image"=w527) -> ("error out"=w526:errorcluster, "Image Pixels (U8)"=w525:u8[][])  [unwired: 2 in, 3 out]
    n134 = Greater Or Equal?(x=w505, y=w504) -> (x >= y?=w502:bool)
    n135 = call <vilib>:"Calculate Frames per Second.vi"("Update Interval (ms)"=u32 2000, "Buffer Number"=w507) -> ("Processed Frames/s"=→"Actual WhiskCam\nFrame Rate":dbl)  [unwired: 7 in, 2 out]
    n136 = local read "CBV Camera"() -> (w499:bool)
    n137 = Write to Binary File(file (use dialog)=w514, data=w525, error in=w526, 5:FALSE ("prepend array or string size? (T)"), 9:T11."little-endian" ("byte order (0:big-endian, network order)")) -> (refnum out=w518:refnum<file>, error out=w509:errorcluster)  [unwired: 1 in, 1 out]
    n138 = local read "Stop"() -> (w501:bool)
    n139 = Unbundle By Name(w509) -> ("status"=w503:bool)
    n140 = Compound Arithmetic op=OR(w503, w502, w501, w499) -> (w500:bool)
    "Whisker Camera" <- w500
  }
  n141 = while {
    tunnel: w268 -> [w573]
    tunnel: w266 -> [w574]
    tunnel: [w530] -> w315
    tunnel: [w565] -> w316
    tunnel: [w564] -> w314
    tunnel: [w558] -> w264
    tunnel: w263 -> [w558]
    tunnel: [w557] -> w262
    tunnel: w261 -> [w557]
    tunnel: w260 -> [w556]
    tunnel: w257 -> [w555]
    tunnel: w256 -> [w554]
    tunnel: w254 -> [w552]
    tunnel: w184 -> [w550]
    tunnel: w183 -> [w549]
    tunnel: [w548] -> w182
    tunnel: [w547] -> w181
    tunnel: w178 -> [w541]
    tunnel: w175 -> [w540]
    tunnel: w171 -> [w538]
    tunnel: w168 -> [w536]
    tunnel: w166 -> [w546]
    tunnel: w155 -> [w539]
    tunnel: w100 -> [w543]
    tunnel: w37 -> [w532]
    tunnel: [w532] -> w36
    tunnel: [w531] -> w34
    tunnel: w35 -> [w531]
    i -> [w572]
    stop <- w534 stop-if-true
    # "Track Time elapsed during trial"
    # "Write T/F \nto Solenoid\nArray"
    # "Track ISI"
    n142 = Tick Count (ms)() -> (millisecond timer value=w562:u32)
    n143 = call <vilib>:"IMAQ Extract Buffer.vi"("error in (no error)"=w574, "Buffer to extract"=w572, "IMAQ Session In"=w573) -> ("error out"=w563:errorcluster, "Buffer Number"=w542:i32, "Image Out"=w570:T4, "IMAQ Session Out"=w565:refnum<k11>)  [unwired: 5 out]
    "Last CBV\nBuffer" <- w542
    n144 = case shown="True" w543 {
      selector: w543 -> [w576 _]
      tunnel: w542 -> [_ w586]
      tunnel: w541 -> [_ w585]
      tunnel: w540 -> [_ w584]
      tunnel: w539 -> [_ w583]
      tunnel: w538 -> [_ w580]
      tunnel: [0.0 ("element") w577] -> w537
      tunnel: w536 -> [_ w579]
      tunnel: [w576 w578] -> w535
      frame False {
      }
      frame True {
        # "Track Solenoid\nOrder"
        # "Track ISI"
        n145 = Quotient & Remainder(x=w586, y=w585) -> (x-y*floor(x/y)=w588:dbl, floor(x/y)=w581:dbl)
        n146 = Add(x=w584, y=w583) -> (x+y=w587:dbl)
        n147 = Quotient & Remainder(x=w581, y=w580) -> (x-y*floor(x/y)=w582:dbl)  [unwired: 1 out]
        n148 = Index Array(array=w579, index=w582) -> (element=w577:dbl)
        n149 = In Range and Coerce(upper limit=w587, x=w588, lower limit=w583) -> (In Range?=w578:bool)  [unwired: 1 out]
      }
    }
    n150 = Subtract(x=w562, y=w556) -> (x-y=w561:u32)
    n151 = local write "Stop"("Stop") -> ()
    n152 = Multiply(x=w561, y=1.667e-05) -> (x*y=w560:dbl)
    n153 = call "IMAQ ImageToArray"("error in (no error)"=w563, "Image"=w570) -> ("error out"=w569:errorcluster, "Image Pixels (I16)"=w568:i16[][])  [unwired: 2 in, 3 out]
    n154 = call <vilib>:"Calculate Frames per Second.vi"("Update Interval (ms)"=u32 2000, "Buffer Number"=w542) -> ("Processed Frames/s"=→"Actual CBVCam\nFrame Rate":dbl)  [unwired: 7 in, 2 out]
    n155 = Greater Or Equal?(x=w542, y=w555) -> (x >= y?=w559:bool)
    n156 = Bundle("Recording Time (min)"=w554, w560) -> (→"Trial Time Elapsed (Min)":cluster{"Recording Time (min)":dbl, dbl})  [unwired: 1 in]
    n157 = Write to Binary File(file (use dialog)=w552, data=w568, error in=w569, 5:FALSE ("prepend array or string size? (T)"), 9:T11."big-endian, network order" ("byte order (0:big-endian, network order)")) -> (refnum out=w564:refnum<file>, error out=w530:errorcluster)  [unwired: 1 in, 1 out]
    n158 = Compound Arithmetic op=OR(w530, "Stop", w559) -> (w534:bool)
    "CBV Camera" <- w534
    n159 = Replace Array Subset(array=w546, new element=w535, index=w537) -> (w545:bool[])
    "Solenoids" <- w545
    n160 = call-poly <vilib>:"DAQmx Write.vi"("task/channels in"=w550, "data"=w545, "error in"=w549) -> ("task out"=w548:refnum<k21>, "error out"=w547:errorcluster)  [unwired: 10 in, 1 out]
  }
  n161 = while {
    tunnel: w302 -> [w598]
    tunnel: w296 -> [w596]
    tunnel: w294 -> [w595]
    tunnel: w292 -> [w594]
    tunnel: w289 -> [w590]
    tunnel: [w592] -> w288
    tunnel: [w591] -> w286
    tunnel: [w590] -> w287
    stop <- w601 stop-if-true
    n162 = Tick Count (ms)() -> (millisecond timer value=w602:u32)
    n163 = Subtract(x=w602, y=w598) -> (x-y=w603:u32)
    n164 = Divide(x=w603, y=u32 1000) -> (x/y=w597:dbl)
    n165 = call "WebCam Grab_atw1.vi"("Session In"=w595, "Image In"=w596, "Trial Time"=w597, "AVI Refnum"=w590, "error in"=w594) -> ("Session Out"=w592:T1, "WebCam Img Out"=→"WebCam":T4, "Buffer Number Out"=w589:u32, "error out"=w591:errorcluster)  [unwired: 7 in]
    n166 = local read "CBV Camera"() -> (w601:bool)
    n167 = call <vilib>:"Calculate Frames per Second.vi"("Update Interval (ms)"=u32 5000, "Buffer Number"=w589) -> ("Processed Frames/s"=→"Actual WebCam Frame Rate":dbl)  [unwired: 7 in, 2 out]
  }
  n168 = call <vilib>:"DAQmx Stop Task.vi"("task/channels in"=w182, "error in"=w181) -> ("task out"=w180:refnum<k21>, "error out"=w179:errorcluster)  [unwired: 12 in]
  n169 = call-poly <vilib>:"DAQmx Write.vi"("task/channels in"=w36, "data"=FALSE, "error in"=w34) -> ("task out"=w33:refnum<k21>, "error out"=w31:errorcluster)  [unwired: 10 in, 1 out]
  n170 = call <vilib>:"DAQmx Stop Task.vi"("task/channels in"=w264, "error in"=w262) -> ()  [unwired: 12 in, 2 out]
  n171 = call <vilib>:"DAQmx Stop Task.vi"("task/channels in"=w282, "error in"=w284) -> ()  [unwired: 12 in, 2 out]
  n172 = Close File(refnum=w281, error in=w157) -> (path=w212:path, error out=w211:errorcluster)
  n173 = call <vilib>:"IMAQdx Close Camera.vi"("error in"=w286, "Session In"=w288) -> ()  [unwired: 9 in, 1 out]
  n174 = call "IMAQ AVI2 Close"("error in (no error)"=w286, "AVI Refnum"=w287) -> ("error out"=w214:errorcluster)  [unwired: 9 in]
  n175 = call <vilib>:"DAQmx Stop Task.vi"("task/channels in"=w235, "error in"=w71) -> ("task out"=w159:refnum<k21>, "error out"=w158:errorcluster)  [unwired: 12 in]
  n176 = call <vilib>:"DAQmx Stop Task.vi"("task/channels in"=w33, "error in"=w31) -> ("task out"=w32:refnum<k21>, "error out"=w30:errorcluster)  [unwired: 12 in]
  n177 = call <vilib>:"IMAQdx Close Camera.vi"("error in"=w157, "Session In"=w68) -> ()  [unwired: 9 in, 1 out]
  n178 = call <vilib>:"DAQmx Clear Task.vi"("task in"=w180, "error in"=w179) -> ()  [unwired: 13 in, 1 out]
  n179 = call <vilib>:"DAQmx Clear Task.vi"("task in"=w159, "error in"=w158) -> ()  [unwired: 13 in, 1 out]
  n180 = Delete From Array(array=w57, length=1, index=0) -> (array with subset deleted=w1:u32[])  [unwired: 1 out]
  n181 = call <vilib>:"DAQmx Clear Task.vi"("task in"=w32, "error in"=w30) -> ()  [unwired: 13 in, 1 out]
  n182 = Delete From Array(array=w221, length=1, index=0) -> (array with subset deleted=w2:u32[])  [unwired: 1 out]
  n183 = call <vilib>:"IMAQ Extract Buffer.vi"("error in (no error)"=w315, "Buffer to extract"=-1, "IMAQ Session In"=w316) -> ("error out"=w338:errorcluster, "IMAQ Session Out"=w337:refnum<k11>)  [unwired: 7 out]
  n184 = Close File(refnum=w314) -> (path=w215:path)  [unwired: 1 in, 1 out]
  n185 = Build Array(w1, w2) -> (w5:u32[][])
  n186 = call <vilib>:"IMAQ Close.vi"("error in (no error)"=w338, "IMAQ Session In"=w337) -> ("error out"=w340:errorcluster)  [unwired: 9 out]
  n187 = Array To Spreadsheet String(delimiter (Tab)=",", array=w1, 3:"%d" ("format string")) -> (spreadsheet string=w62:string)
  n188 = Array To Spreadsheet String(delimiter (Tab)=",", array=w2, 3:"%d" ("format string")) -> (spreadsheet string=w61:string)
  n189 = call <vilib>:"Trim Whitespace.vi"("string"=w61) -> ("trimmed string"=w60:string)  [unwired: 1 in]
  n190 = call <vilib>:"Trim Whitespace.vi"("string"=w62) -> ("trimmed string"=w59:string)  [unwired: 1 in]
  n191 = Transpose 2D Array(2D array=w5) -> (transposed array=w4:u32[][])
  n192 = for {
    N: w156 -> [_]
    tunnel: w333 -> [w608] mode=indexing
    shift-right: [w606] -> w217
    shift-left: w340 -> [w607]
    n193 = call "IMAQ Dispose"("All Images? (No)"=FALSE, "Image"=w608, "error in (no error)"=w607) -> ("error out"=w606:errorcluster)  [unwired: 3 out]
  }
  n194 = Build Array(w59, w60) -> (w58:string[])
  n195 = Number To Decimal String(number=w4) -> (decimal integer string=→"Dropped Frame Table":string[][])  [unwired: 1 in]
  n196 = TDMS Set Properties(5:w58, 7:string[] ["WhiskerCam_DroppedFrameIndex", "WhiskerCam_NumberDropped"] ("channel name(s) in (Untitled)"), 8:w71, 11:w72) -> (0:w70:errorcluster, 3:w67:refnum<k34>)  [unwired: 2 in, 2 out]
  n197 = TDMS Close(8:w70, 11:w67) -> (0:w218:errorcluster, 3:w205:path)
  n198 = TDMS Defragment(4:w218, 7:w205) -> (0:w201:errorcluster)
  n199 = Path To String(path=w205) -> (string=w207:string)
  n200 = Concatenate Strings(w207, "_index" ("string")) -> (w204:string)
  n201 = String To Path(string=w204) -> (path=w203:path)
  n202 = Move(source path=w215, error in=w217, 10:"Target Path") -> (error out=w216:errorcluster)  [unwired: 2 in, 2 out]
  n203 = Move(source path=w203, error in=w201, 10:"Target Path") -> ()  [unwired: 2 in, 3 out]
  n204 = Move(source path=w205, error in=w201, 10:"Target Path") -> (error out=w210:errorcluster)  [unwired: 2 in, 2 out]
  n205 = Move(source path=w212, error in=w211, 10:"Target Path") -> (error out=w209:errorcluster)  [unwired: 2 in, 2 out]
  n206 = Move(source path=w213, error in=w214, 10:"Target Path") -> (error out=w208:errorcluster)  [unwired: 2 in, 2 out]
  n207 = call <vilib>:"Simple Error Handler.vi"("error in (no error)"=w216) -> ()  [unwired: 1 in, 8 out]
  n208 = call <vilib>:"Simple Error Handler.vi"("error in (no error)"=w210) -> ()  [unwired: 1 in, 8 out]
  n209 = call <vilib>:"Simple Error Handler.vi"("error in (no error)"=w209) -> ()  [unwired: 1 in, 8 out]
  n210 = call <vilib>:"Simple Error Handler.vi"("error in (no error)"=w208) -> ()  [unwired: 1 in, 8 out]
